vi "readU32.vi"(8 "error in (no error)":errorcluster, 11 "ModbusBuffer in":refnum<class "ModbusBufferBuilder.lvclass">) -> (0 "error out":errorcluster, 2 "Output":u32, 3 "ModbusBuffer out":refnum<class "ModbusBufferBuilder.lvclass">)   [LabVIEW 2016, in "ModbusBufferBuilder.lvclass"]
uses:
  ModbusBufferBuilder.lvclass
  ModbusBufferBuilder.lvclass/ModbusBufferBuilder.ctl
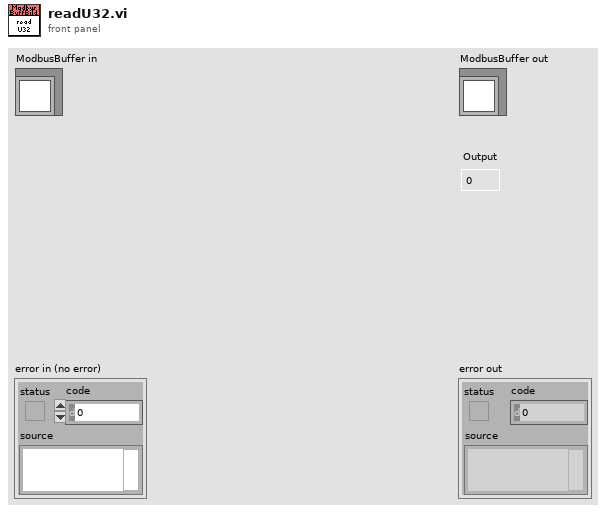
[diagram p1: front panel]
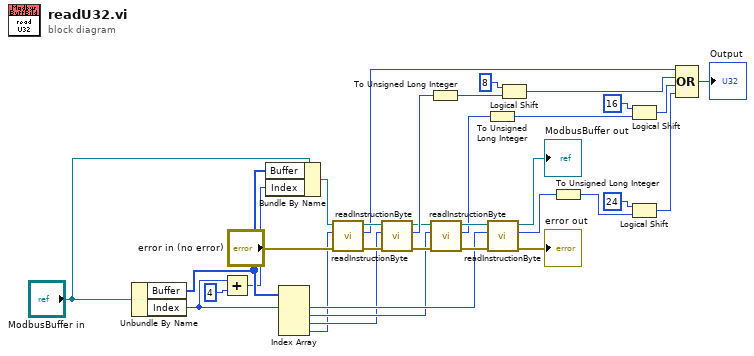
[diagram p0: block diagram]
diagram:
  n1 = Unbundle By Name("ModbusBuffer in") -> ("Buffer"=w32:u16[], "Index"=w29:i32)
  n2 = Add(x=w29, y=4) -> (x+y=w27:i32)
  n3 = Bundle By Name(cluster="ModbusBuffer in", "Buffer"=w32, "Index"=w27) -> (w31:refnum<class "ModbusBufferBuilder.lvclass">)
  n4 = Index Array(array=w32, index #1=w29) -> (element #1=w4:u16, element #2=w3:u16, element #3=w2:u16, element #4=w1:u16)  [unwired: 3 in]
  n5 = call "readInstructionByte.vi"("error in (no error)"="error in (no error)", "Instruction"=w1, "ModbusBuffer in"=w31) -> ("error out"=w24:errorcluster, "Output"=w25:u8, "ModbusBuffer out"=w26:refnum<class "ModbusBufferBuilder.lvclass">)  [unwired: 6 in]
  n6 = call "readInstructionByte.vi"("error in (no error)"=w24, "Instruction"=w2, "ModbusBuffer in"=w26) -> ("error out"=w15:errorcluster, "Output"=w20:u8, "ModbusBuffer out"=w18:refnum<class "ModbusBufferBuilder.lvclass">)  [unwired: 6 in]
  n7 = To Unsigned Long Integer(number=w20) -> (unsigned 32bit integer=w19:u32)
  n8 = call "readInstructionByte.vi"("error in (no error)"=w15, "Instruction"=w3, "ModbusBuffer in"=w18) -> ("error out"=w14:errorcluster, "Output"=w8:u8, "ModbusBuffer out"=w17:refnum<class "ModbusBufferBuilder.lvclass">)  [unwired: 6 in]
  n9 = To Unsigned Long Integer(number=w8) -> (unsigned 32bit integer=w12:u32)
  n10 = call "readInstructionByte.vi"("error in (no error)"=w14, "Instruction"=w4, "ModbusBuffer in"=w17) -> ("error out"=→"error out":errorcluster, "Output"=w7:u8, "ModbusBuffer out"=→"ModbusBuffer out":refnum<class "ModbusBufferBuilder.lvclass">)  [unwired: 6 in]
  n11 = Logical Shift(y=i16 8, x=w19) -> (x << y=w22:u32)
  n12 = To Unsigned Long Integer(number=w7) -> (unsigned 32bit integer=w9:u32)
  n13 = Logical Shift(y=i16 16, x=w12) -> (x << y=w5:u32)
  n14 = Logical Shift(y=i16 24, x=w9) -> (x << y=w6:u32)
  n15 = Compound Arithmetic op=OR(w25, w22, w5, w6) -> (→"Output":u32)
